vi "REV2_Read_Stat.vi"(8 "error in (no error)":errorcluster, 9 "Stat Address":T1[](array[typedef]) items=["Torque Enable", "Homing Complete", "Goal Id", "Goal Iq", "Goal Velo", "Goal Posi", "Present Id", "Present Iq", "Present Velo", "Present Posi", "Bus Voltage", "Temperature Winding", "Temperature MOSFET", "Temperature IC", "Error Status", "Iq_Temps"], 10 "ID":u8, 11 "VISA Refnum in":refnum<visa-resource-name>) -> (0 "error out":errorcluster, 1 "ERROR":u8, 2 "Data":dbl[](array[numeric]), 3 "VISA Refnum out":refnum<visa-resource-name>)   [LabVIEW 2016, in "REV_2.lvlib"]
uses:
  REV_2.lvlib
  REV2_Instructions.ctl
  REV2_Stat_Addr.ctl
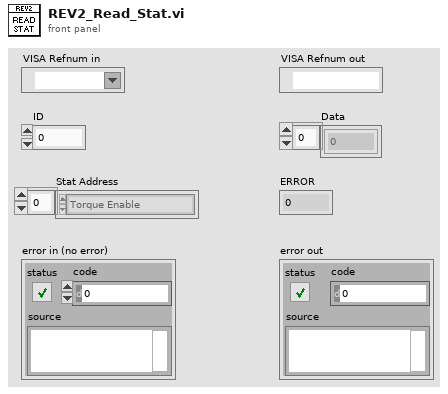
[diagram p1: front panel]
types:
  T1 = typedef "REV_2.lvlib/REV2_Stat_Addr.ctl" = u8
  T2 = enum16{"big-endian, network order", "native, host order", "little-endian"}
  T3 = typedef "REV_2.lvlib/REV2_Instructions.ctl" = u8
  T4 = cluster{"ID":u8, "ERROR":u8, "ChechSumError?":bool, "Data":string}
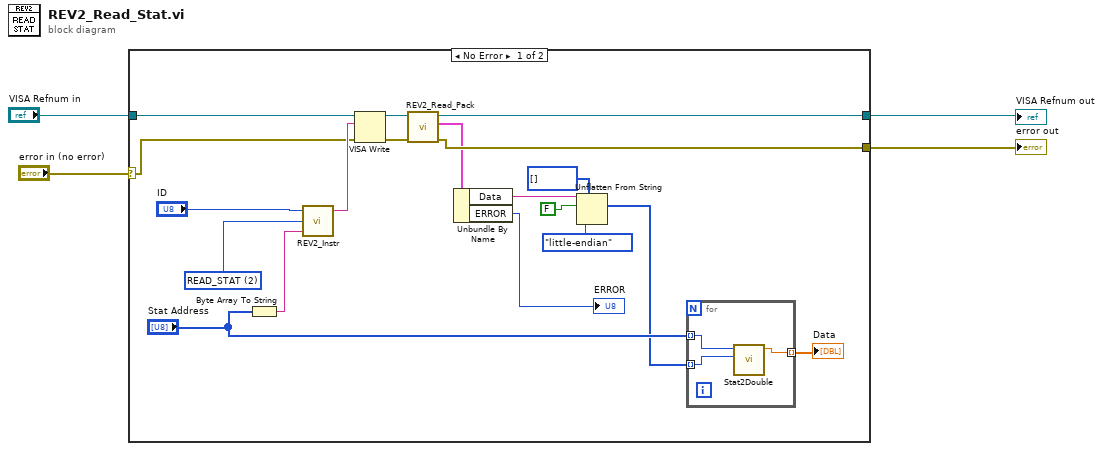
[diagram p0: block diagram]
diagram:
  n1 = case shown="No Error" "error in (no error)" {
    selector: "error in (no error)" -> [w5 w28]
    tunnel: [w16 w27] -> w4
    tunnel: [w15 w28] -> w3
    tunnel: "VISA Refnum in" -> [w9 w27]
    frame No Error {
      w18 = T3 2 items=["PING"=1, "READ_STAT"=2, "WRITE_STAT"=3, "READ_CONFIG"=4, "WRITE_CONFIG"=5, "SAVE_CONFIG"=6] ("Instruction")
      n2 = Byte Array To String(unsigned byte array="Stat Address") -> (string=w17:string)
      n3 = call "REV2_Instr.vi"("Parameter"=w17, "Instruction"=w18, "ID"="ID") -> ("Output"=w11:string)  [unwired: 2 in]
      n4 = VISA Write(VISA resource name=w9, write buffer=w11, error in (no error)=w5) -> (VISA resource name out=w13:refnum<visa-resource-name>, error out=w14:errorcluster)  [unwired: 1 out]
      n5 = call "REV2_Read_Pack.vi"("error in (no error)"=w14, "VISA Refnum in"=w13) -> ("error out"=w15:errorcluster, "output cluster"=w12:T4, "VISA Refnum out"=w16:refnum<visa-resource-name>)  [unwired: 7 in]
      n6 = Unbundle By Name(w12) -> ("Data"=w23:string, "ERROR"=→"ERROR":u8)
      n7 = Unflatten From String(type=u32[] [], binary string=w23, data includes array or string size? (T)=FALSE, byte order (0:big-endian, network order)=T2."little-endian") -> (value=w7:u32[])  [unwired: 1 in, 2 out]
      n8 = for {
        tunnel: "Stat Address" -> [w26] mode=indexing
        tunnel: w7 -> [w25] mode=indexing
        tunnel: [w24] -> w6 mode=indexing
        n9 = call "Stat2Double.vi"("Numeric in"=w25, "Stat Address"=w26) -> ("Numeric out"=w24:dbl)  [unwired: 9 in]
      }
      "Data" <- w6
    }
    frame Error {
    }
  }
  "VISA Refnum out" <- w4
  "error out" <- w3
